vi "sign.vi"(8 "Error In":errorcluster, 11 "number in":i32) -> (0 "Error Out":errorcluster, 3 "number out":i32)   [LabVIEW 2014]
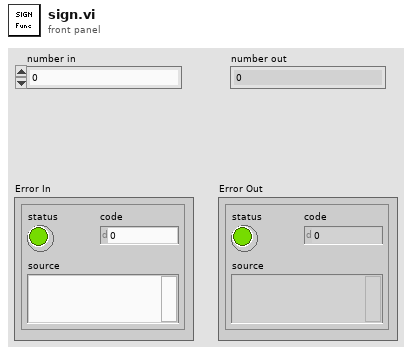
[diagram p1: front panel]
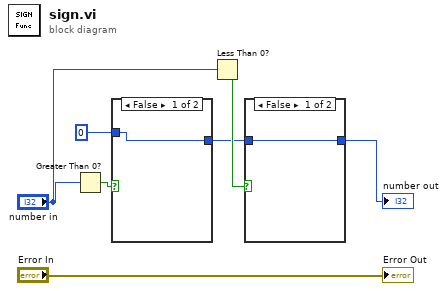
[diagram p0: block diagram]
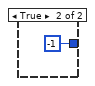
[diagram p2: hidden frame]
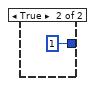
[diagram p3: hidden frame]
diagram:
  n1 = Greater Than 0?(x="number in") -> (x > 0?=w6:bool)
  n2 = case shown="False" w6 {
    tunnel: 0 -> [w8 _]
    tunnel: [w8 1] -> w1
    frame False {
    }
    frame True {
    }
  }
  n3 = Less Than 0?(x="number in") -> (x < 0?=w5:bool)
  n4 = case shown="False" w5 {
    tunnel: [w10 -1] -> w3
    tunnel: w1 -> [w10 _]
    frame False {
    }
    frame True {
    }
  }
  "number out" <- w3
  "Error Out" <- "Error In"
